vi "Keysight5700 Main.vi"() -> ()   [LabVIEW 2021]
uses:
  Controls/PS States.ctl
panel:
  out "Connect?":bool
  in  "stop":bool
  in  "Measurement Type":i32(ring)=1 items=["Current", "Voltage", "Power"]
  out "error out":errorcluster
  out "Measurement":dbl=nan
  in  "Enable Output":bool=TRUE
  in  "Alias":string="PS4"
  in  "Setting":T1={"Max Volt"=10.0, "Voltage Set"=5.0, "Current Lim"=0.5}
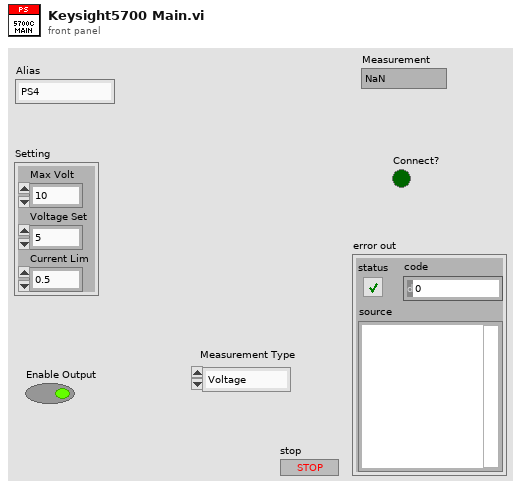
[diagram p1: front panel]
types:
  T1 = cluster{"Max Volt":dbl, "Voltage Set":dbl, "Current Lim":dbl}
  T2 = typedef "PS States.ctl" = enum16{"Init", "Config", "Enable Output", "Measure", "Close"}
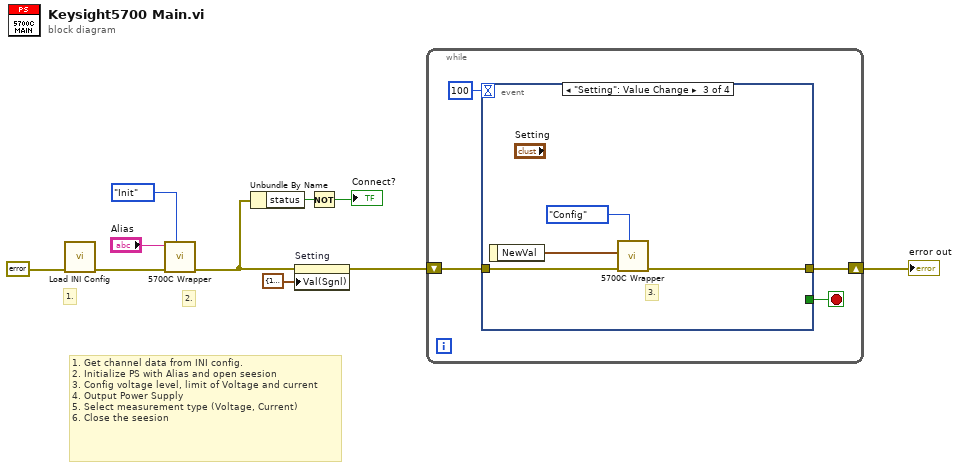
[diagram p0: block diagram]
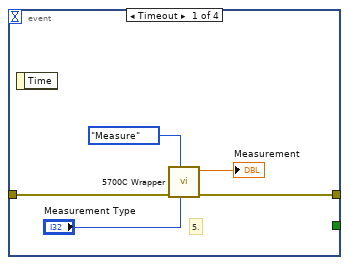
[diagram p2: hidden frame]
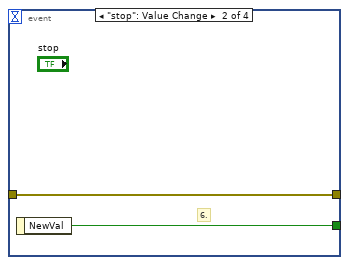
[diagram p3: hidden frame]
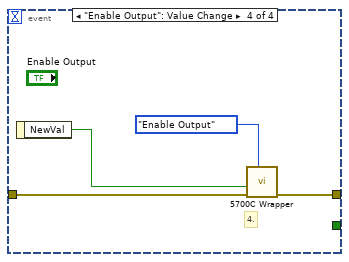
[diagram p4: hidden frame]
diagram:
  # "1. Get channel data from INI config.\n2. Initialize PS with Alias and open seesion \n3. Config voltage level, limit of Voltage and current\n4. Output Power Supply\n5. Select measurement type (Voltage, Current)\n6. Close the seesion"
  # "2."
  # "1."
  n1 = call "Load INI Config.vi"("error in"=errorcluster {"status"=FALSE, "code"=0, "source"=""}) -> ("error out"=w7:errorcluster)  [unwired: 10 in]
  n2 = call "5700C Wrapper.vi"("States"=PS_States."Init", "error in"=w7, "Alias"="Alias") -> ("error out"=w3:errorcluster)  [unwired: 5 in, 3 out]
  n3 = Unbundle By Name(w3) -> ("status"=w4:bool)
  n4 = property on="Setting" class="Clust (strict)"(error in=w3, "Val(Sgnl)"=T1 {"Max Volt"=10.0, "Voltage Set"=5.0, "Current Lim"=0.5} ("Value (Signaling)")) -> (error out=w2:errorcluster)  [unwired: 1 in, 1 out]
  n5 = Not(x=w4) -> (.not. x?=→"Connect?":bool)
  n6 = while {
    shift-right: [w12] -> w6
    shift-left: w2 -> [w13]
    stop <- w14 stop-if-true
    n7 = event shown="[2] \"Setting\": Value Change" {
      selector: _ -> [_ _ _ _]
      dyn-events: _ -> [_ _ _ _]
      timeout: 100 -> [_ _ _ _]
      tunnel: [_ w21 _ _] -> w14
      tunnel: [w17 w20 w24 w28] -> w12
      tunnel: w13 -> [w19 w20 w25 w29]
      event Timeout {
        # "5."
        n8 = event-data() -> ()  [unwired: 1 in, 1 out]
        n9 = call "5700C Wrapper.vi"("Measurement Type"="Measurement Type", "States"=PS_States."Measure", "error in"=w19) -> ("error out"=w17:errorcluster, "Measurement"=→"Measurement":dbl)  [unwired: 5 in, 2 out]
      }
      event "stop": Value Change {
        # "6."
        n10 = event-data() -> ("NewVal"=w21:bool)  [unwired: 1 in]
      }
      event "Setting": Value Change {
        # "3."
        n11 = event-data() -> ("NewVal"=w23:T1)  [unwired: 1 in]
        n12 = call "5700C Wrapper.vi"("States"=PS_States."Config", "error in"=w25, "Setting"=w23) -> ("error out"=w24:errorcluster)  [unwired: 5 in, 3 out]
      }
      event "Enable Output": Value Change {
        # "4."
        n13 = event-data() -> ("NewVal"=w26:bool)  [unwired: 1 in]
        n14 = call "5700C Wrapper.vi"("States"=PS_States."Enable Output", "error in"=w29, "Enable Output"=w26) -> ("error out"=w28:errorcluster)  [unwired: 5 in, 3 out]
      }
    }
  }
  "error out" <- w6
